vi "Shooter and Accelerator.vi"(8 "error in (no error)":errorcluster, 9 "Shooting Overide?":bool, 10 "Shooting Position":T1=enum."Front", 11 "Power Cell Handler in":refnum<class "Power Cell Handler.lvclass">) -> (0 "error out":errorcluster, 2 "Ready to fire":bool, 3 "Power Cell Handler out":refnum<class "Power Cell Handler.lvclass">)   [LabVIEW 2019, in "Power Cell Handler.lvlib" / "Power Cell Handler.lvclass"]
uses:
  Power Cell Handler.lvclass
  Controls/Shooting Position.ctl
  <vilib>/Rock Robotics/WPI/ThirdParty/Phoenix-LabVIEW/Motor Controller/Controls/CTRE_Phoenix_MotorControl_ControlMode.ctl
  Power Cell Handler.lvclass/Power Cell Handler.ctl
  <vilib>/Rock Robotics/Network Tables/NT Read Number.vi
  <vilib>/Rock Robotics/WPI/ThirdParty/Phoenix-LabVIEW/Motor Controller/Get/CTRE_Phoenix_MotorController_GetClosedLoopData.vi
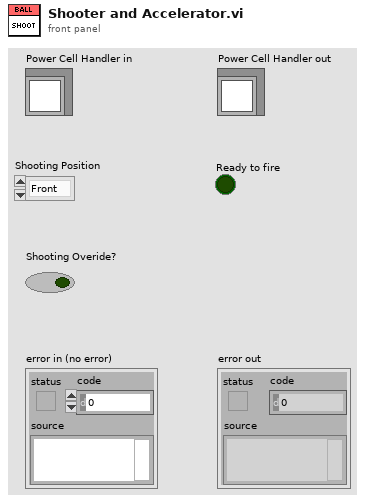
[diagram p1: front panel]
types:
  T1 = typedef "Power Cell Handler.lvlib/Power Cell Handler.lvclass/Shooting Position.ctl" = enum16{"Rest", "Front", "Middle", "Back"}
  T2 = typedef "CTRE_Phoenix_MotorControl_ControlMode.ctl" = u16
  T3 = typedef "WPI_MotorControlDeviceRef.ctl" = cluster{"DeviceStatus":errorcluster, "Type":T4, "PWM":cluster{"PWM Channel":T5, "DeadBand":T6}, "CAN":cluster{"Device Number":u8, "SetOutput VI Ref":variant, "GetOutput VI Ref":variant, "Enable VI Ref":variant, "Disable VI Ref":variant, "Data":variant}, "Invert":bool, "DIO PWM":cluster{"PWM \"Enable\" Channel":T5, "DIOChannel":T7, "PWM Rate":dbl}}
  T4 = typedef "WPI_MotorControlType.ctl" = enum16{"PWM", "CAN", "DIO PWM"}
  T5 = typedef "FPGA_DIOPWMChannel.ctl" = enum8{"PWM 0", "PWM 1", "PWM 2", "PWM 3", "PWM 4", "PWM 5", "PWM 6", "PWM 7", "PWM 8", "PWM 9", "PWM MXP 0", "PWM MXP 1", "PWM MXP 2", "PWM MXP 3", "PWM MXP 4", "PWM MXP 5", "PWM MXP 6", "PWM MXP 7", "PWM MXP 8", "PWM MXP 9", "Invalid"}
  T6 = typedef "WPI_PWMDeadband.ctl" = cluster{"Name":string, "maxPositivePwm":i32, "minPositivePwm":i32, "centerPwm":i32, "maxNegativePwm":i32, "minNegativePwm":i32, "angularRange":u16}
  T7 = typedef "FPGA_DIOChannel.ctl" = enum8{"DIO 0", "DIO 1", "DIO 2", "DIO 3", "DIO 4", "DIO 5", "DIO 6", "DIO 7", "DIO 8", "DIO 9", "DIO MXP 0", "DIO MXP 1", "DIO MXP 2", "DIO MXP 3", "DIO MXP 4", "DIO MXP 5", "DIO MXP 6", "DIO MXP 7", "DIO MXP 8", "DIO MXP 9", "DIO MXP 10", "DIO MXP 11", "DIO MXP 12", "DIO MXP 13", "DIO MXP 14", "DIO MXP 15", "SPI Port CS1", "SPI Port CS2", "SPI Port CS3", "SPI Port MISO", "SPI Port MOSI", "Invalid"}
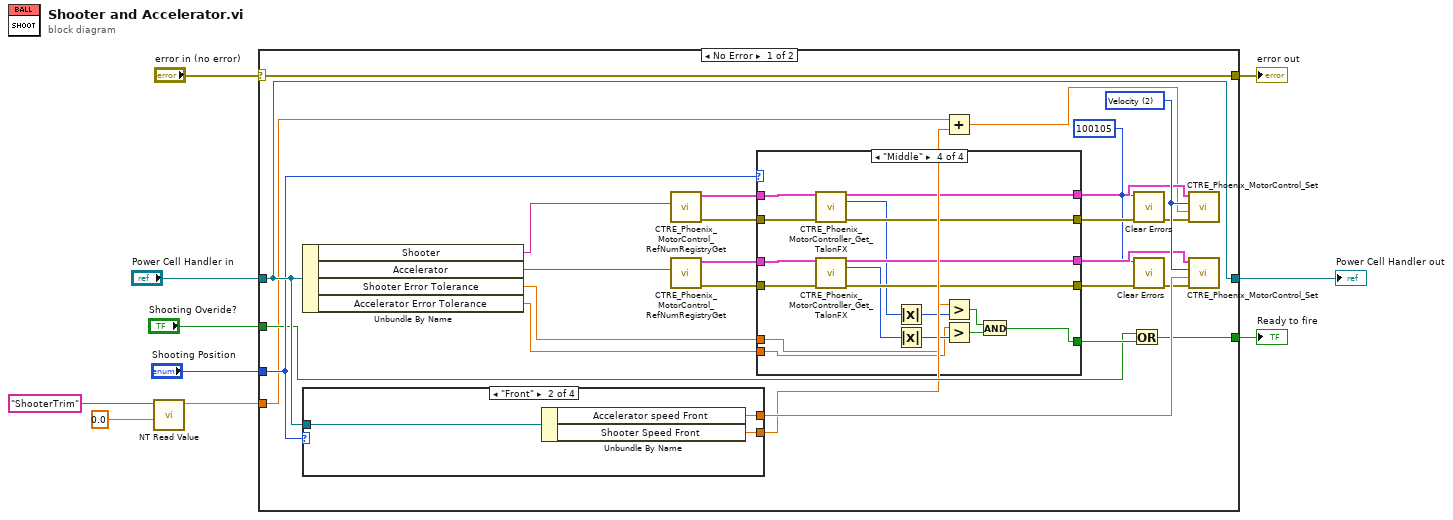
[diagram p0: block diagram]
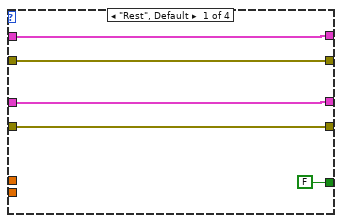
[diagram p2: hidden frame]
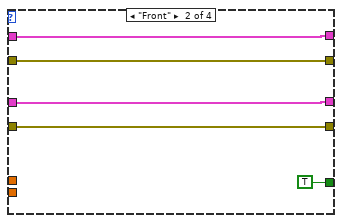
[diagram p3: hidden frame]
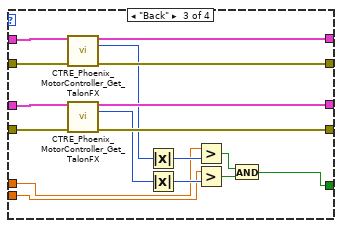
[diagram p4: hidden frame]
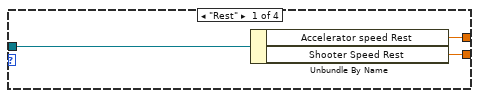
[diagram p5: hidden frame]
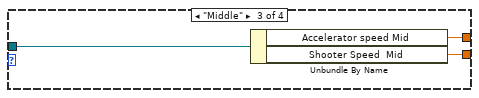
[diagram p6: hidden frame]
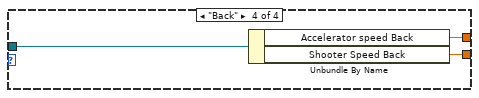
[diagram p7: hidden frame]
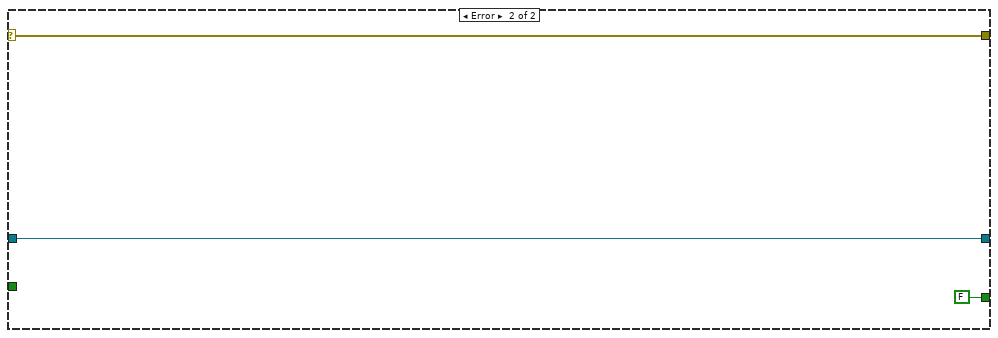
[diagram p8: hidden frame]
diagram:
  n1 = call-poly <vilib>:"NT Read Value.vi"("Default Value"=0.0, "Name"="ShooterTrim") -> ("Numeric"=w3:dbl)  [unwired: 8 in, 1 out]
  n2 = case shown="No Error" "error in (no error)" {
    selector: "error in (no error)" -> [w36 w95]
    tunnel: [w36 w95] -> w9
    tunnel: "Power Cell Handler in" -> [w32 w94]
    tunnel: [w32 w94] -> w7
    tunnel: "Shooting Position" -> [w28 _]
    tunnel: [w26 FALSE] -> w4
    tunnel: "Shooting Overide?" -> [w25 _]
    tunnel: w3 -> [w11 _]
    frame No Error {
      w14 = 100105 ("specific error code to clear (0: all)")
      w31 = T2 2 items=["PercentOutput"=0, "Position"=1, "Velocity"=2, "Current"=3, "Follower"=5, "MotionProfile"=6, "MotionMagic"=7, "MotionProfileArc"=10, "Disabled"=15] ("Control Mode")
      n3 = Unbundle By Name(w32) -> ("Shooter"=w35:string, "Accelerator"=w34:string, "Shooter Error Tolerance"=w15:dbl, "Accelerator Error Tolerance"=w16:dbl)
      n4 = case shown="\"Front\"" w28 {
        tunnel: [w81 w84 w87 w90] -> w13
        tunnel: [w82 w85 w88 w91] -> w33
        tunnel: w32 -> [w83 w86 w89 w92]
        frame "Rest" {
          n5 = Unbundle By Name(w83) -> ("Accelerator speed Rest"=w82:dbl, "Shooter Speed Rest"=w81:dbl)
        }
        frame "Front" {
          n6 = Unbundle By Name(w86) -> ("Accelerator speed Front"=w85:dbl, "Shooter Speed Front"=w84:dbl)
        }
        frame "Middle" {
          n7 = Unbundle By Name(w89) -> ("Accelerator speed Mid"=w88:dbl, "Shooter Speed  Mid"=w87:dbl)
        }
        frame "Back" {
          n8 = Unbundle By Name(w92) -> ("Accelerator speed Back"=w91:dbl, "Shooter Speed Back"=w90:dbl)
        }
      }
      n9 = call <vilib>:"CTRE_Phoenix_MotorControl_RefNumRegistryGet.vi"("refnum name"=w35) -> ("error out"=w22:errorcluster, "PhoenixMotorControlDevRef"=w24:T3)  [unwired: 9 in]
      n10 = call <vilib>:"CTRE_Phoenix_MotorControl_RefNumRegistryGet.vi"("refnum name"=w34) -> ("error out"=w21:errorcluster, "PhoenixMotorControlDevRef"=w23:T3)  [unwired: 9 in]
      n11 = case shown="\"Middle\"" w28 {
        tunnel: [FALSE TRUE w47 w64] -> w27
        tunnel: w24 -> [w40 w45 w63 w80]
        tunnel: w23 -> [w38 w43 w62 w79]
        tunnel: w22 -> [w39 w44 w61 w78]
        tunnel: w21 -> [w37 w42 w60 w77]
        tunnel: [w37 w42 w59 w76] -> w20
        tunnel: [w39 w44 w58 w75] -> w19
        tunnel: [w40 w45 w57 w74] -> w18
        tunnel: [w38 w43 w56 w73] -> w17
        tunnel: w16 -> [_ _ w51 w68]
        tunnel: w15 -> [_ _ w50 w67]
        frame "Rest", Default {
        }
        frame "Front" {
        }
        frame "Back" {
          n12 = call-poly <vilib>:"CTRE_Phoenix_MotorController_Get_TalonFX.vi"("PhoenixMotorControlDevRef"=w63, "error in"=w61) -> ("PhoenixMotorControlDevRef"=w57:T3, "Closed-loop Error"=w49:i32, "error out"=w58:errorcluster)  [unwired: 8 in, 3 out]
          n13 = call-poly <vilib>:"CTRE_Phoenix_MotorController_Get_TalonFX.vi"("PhoenixMotorControlDevRef"=w62, "error in"=w60) -> ("PhoenixMotorControlDevRef"=w56:T3, "Closed-loop Error"=w48:i32, "error out"=w59:errorcluster)  [unwired: 8 in, 3 out]
          n14 = Absolute Value(x=w49) -> (abs(x)=w52:i32)
          n15 = Absolute Value(x=w48) -> (abs(x)=w55:i32)
          n16 = Greater?(x=w50, y=w52) -> (0:w54:bool)
          n17 = Greater?(x=w51, y=w55) -> (0:w53:bool)
          n18 = And(x=w54, y=w53) -> (x .and. y?=w47:bool)
        }
        frame "Middle" {
          n19 = call-poly <vilib>:"CTRE_Phoenix_MotorController_Get_TalonFX.vi"("PhoenixMotorControlDevRef"=w80, "error in"=w78) -> ("PhoenixMotorControlDevRef"=w74:T3, "Closed-loop Error"=w66:i32, "error out"=w75:errorcluster)  [unwired: 8 in, 3 out]
          n20 = call-poly <vilib>:"CTRE_Phoenix_MotorController_Get_TalonFX.vi"("PhoenixMotorControlDevRef"=w79, "error in"=w77) -> ("PhoenixMotorControlDevRef"=w73:T3, "Closed-loop Error"=w65:i32, "error out"=w76:errorcluster)  [unwired: 8 in, 3 out]
          n21 = Absolute Value(x=w66) -> (abs(x)=w69:i32)
          n22 = Absolute Value(x=w65) -> (abs(x)=w72:i32)
          n23 = Greater?(x=w67, y=w69) -> (0:w71:bool)
          n24 = Greater?(x=w68, y=w72) -> (0:w70:bool)
          n25 = And(x=w71, y=w70) -> (x .and. y?=w64:bool)
        }
      }
      n26 = Add(x=w11, y=w13) -> (x+y=w12:dbl)
      n27 = Or(x=w25, y=w27) -> (x .or. y?=w26:bool)
      n28 = call <vilib>:"Clear Errors.vi"("error in (no error)"=w19, "specific error code to clear (0: all)"=w14) -> ("error out"=w29:errorcluster)  [unwired: 4 in, 1 out]
      n29 = call <vilib>:"Clear Errors.vi"("error in (no error)"=w20, "specific error code to clear (0: all)"=w14) -> ("error out"=w30:errorcluster)  [unwired: 4 in, 1 out]
      n30 = call <vilib>:"CTRE_Phoenix_MotorControl_Set.vi"("error in (no error)"=w29, "Output"=w12, "Control Mode"=w31, "PhoenixMotorControlDevRef"=w18) -> ()  [unwired: 6 in, 2 out]
      n31 = call <vilib>:"CTRE_Phoenix_MotorControl_Set.vi"("error in (no error)"=w30, "Output"=w33, "Control Mode"=w31, "PhoenixMotorControlDevRef"=w17) -> ()  [unwired: 6 in, 2 out]
    }
    frame Error {
    }
  }
  "error out" <- w9
  "Power Cell Handler out" <- w7
  "Ready to fire" <- w4
